vi "Win Host - CSV FTR List.vi"(8 "error in (no error)":errorcluster, 11 "Selected Runs?":bool[](array[boolean])) -> (0 "error out":errorcluster, 3 "ftrTypes csv":string)   [LabVIEW 2024]
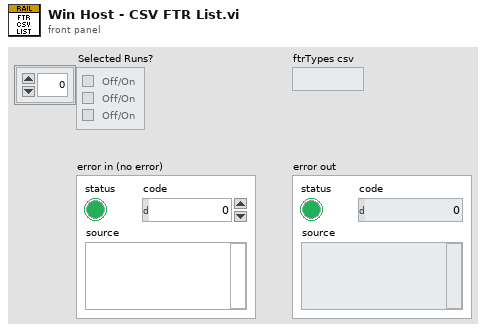
[diagram p1: front panel]
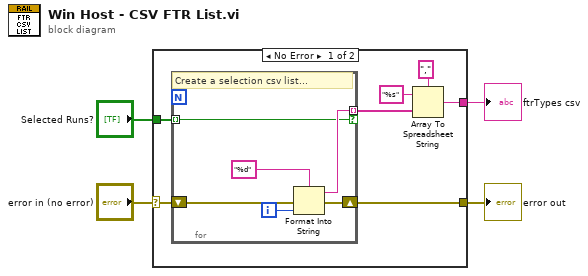
[diagram p0: block diagram]
diagram:
  n1 = case shown="No Error" "error in (no error)" {
    selector: "error in (no error)" -> [w10 w18]
    tunnel: [w9 w18] -> w2
    tunnel: "Selected Runs?" -> [w11 _]
    tunnel: [w6 _] -> w4
    frame No Error {
      n2 = for {
        tunnel: w11 -> [w12] mode=indexing
        shift-right: [w16] -> w9
        shift-left: w10 -> [w17]
        tunnel: [w13] -> w8 mode=indexing if=w12
        i -> [w15]
        # "Create a selection csv list..."
        n3 = Format Into String(format string="%d", error in=w17, w15) -> (resulting string=w13:string, error out=w16:errorcluster)  [unwired: 1 in]
      }
      n4 = Array To Spreadsheet String(delimiter (Tab)=",", array=w8, 3:"%s" ("format string")) -> (spreadsheet string=w6:string)
    }
    frame Error {
    }
  }
  "ftrTypes csv" <- w4
  "error out" <- w2
